vi "Get Workers by Function.vi"(6 "RSVP":bool, 8 "error in (no error)":errorcluster, 9 "Requestor":refnum<class "Message Enqueuer.lvclass">, 10 "Function":string, 11 "Application Controller in":refnum<class "Application Controller.lvclass">) -> (0 "error out":errorcluster, 1 "found":bool, 2 "Workers":string[](array[string]), 3 "Application Controller out":refnum<class "Application Controller.lvclass">)   [LabVIEW 2016, in "Application Controller.lvclass"]
uses:
  Application Controller.lvclass
  <vilib>/ActorFramework/Message Enqueuer/Message Enqueuer.lvclass
  Application Controller.lvclass/Application Controller.ctl
  Sequence Elements/Sequence Element Messages/Workers by Function Response Msg/Workers by Function Response Msg.lvclass/Workers by Function Response Msg.ctl
  <vilib>/ActorFramework/Message Enqueuer/Message Enqueuer.lvclass/Message Enqueuer.ctl
  <vilib>/ActorFramework/Message Enqueuer/Enqueue.vi
  Sequence Elements/Sequence Element Messages/Workers by Function Response Msg/Workers by Function Response Msg.lvclass
  D:/Program Files/National Instruments/LabVIEW 2016/vi.lib/ActorFramework/Message/Message.lvclass
  <vilib>/ActorFramework/Message Priority Queue/Priority Enqueue.vi
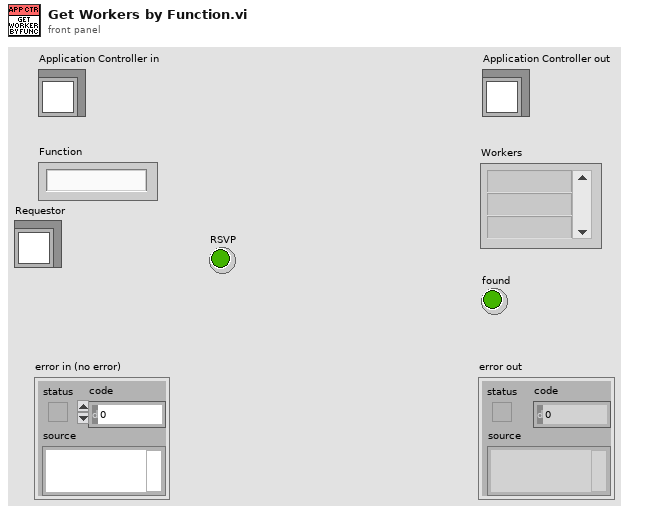
[diagram p1: front panel]
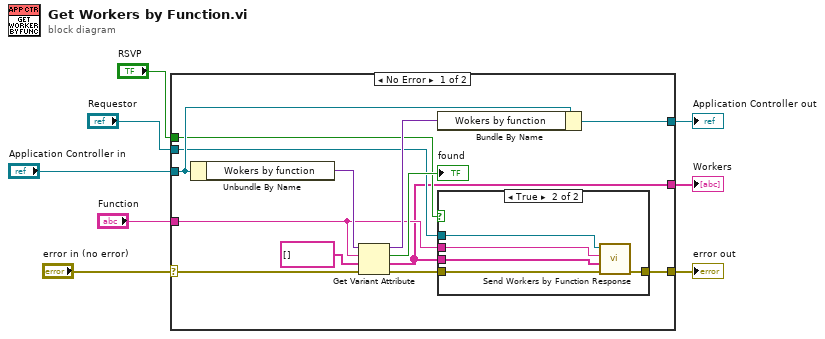
[diagram p0: block diagram]
diagram:
  n1 = case shown="No Error" "error in (no error)" {
    selector: "error in (no error)" -> [w17 w29]
    tunnel: [w12 w29] -> w7
    tunnel: [w18 w28] -> w5
    tunnel: "Application Controller in" -> [w21 w28]
    tunnel: "Function" -> [w10 _]
    tunnel: [w9 _] -> w3
    tunnel: "Requestor" -> [w14 _]
    tunnel: "RSVP" -> [w11 _]
    frame No Error {
      n2 = Unbundle By Name(w21) -> ("Wokers by function"=w20:variant)
      n3 = Get Variant Attribute(Variant=w20, name=w10, default value (empty Variant)=string[] [], error in=w17) -> (duplicate Variant=w16:variant, found=→"found":bool, value=w9:string[], error out=w13:errorcluster)
      n4 = Bundle By Name(cluster=w21, "Wokers by function"=w16) -> (w18:refnum<class "Application Controller.lvclass">)
      n5 = case shown="True" w11 {
        tunnel: w14 -> [_ w27]
        tunnel: w13 -> [w22 w26]
        tunnel: [w22 w25] -> w12
        tunnel: w10 -> [_ w24]
        tunnel: w9 -> [_ w23]
        frame False {
        }
        frame True {
          n6 = call "Send Workers by Function Response.vi"("error in (no error)"=w26, "Workers"=w23, "Function"=w24, "Message Enqueuer"=w27) -> ("error out"=w25:errorcluster)  [unwired: 6 in, 1 out]
        }
      }
    }
    frame Error {
    }
  }
  "error out" <- w7
  "Application Controller out" <- w5
  "Workers" <- w3
